vi "MD5 Padding__ogtk.vi"(1 "String":string) -> (0 "MD5 Padded String":string)   [LabVIEW 2015]
panel:
  # "[OpenG VI Tags] ***Do Not Remove***"
  # "MD5 Padding.vi\n\nDerived from the RSA Data Security, Inc. MD5 Message-Digest Algorithm\n\nPlease visit http://www.OpenG.org to learn about the\nOpen Source LabVIEW software movement.\n\nNOTICE -- YOU MUST LEAVE THIS NOTICE IN PLACE.  PER THE TERMS OF THE LICENSE BELOW, YOU MAY SUBLICENSE THIS SOFTWARE \nIN ANY WAY THAT DOES NOT CONFLICT WITH THIS LICENSE.\n\n### BSD License (http://www.opensource.org/licenses/bsd-license.php) Begin ###\n \nCopyright (c) 2004, Enrique Vargas <vargas@visecurity.com>\n\nAll rights reserved.\n\nRedistribution and use in source and binary forms, with or without modification, are permitted provided that the following conditions are met:\n\n    * Redistributions of source code must retain the above copyright notice, this list of conditions and the following disclaimer.\n    * Redistributions in binary form must reproduce the above copyright notice, this list of conditions and the following disclaimer in the \n       documentation and/or other materials provided with the distribution.\n    * Neither the name of SciWare, James Kring, Inc., nor the names of its contributors may be used to endorse or promote products derived \n       from this software without specific prior written permission.\n\nTHIS SOFTWARE IS PROVIDED BY THE COPYRIGHT HOLDERS AND CONTRIBUTORS \"AS IS\" AND ANY EXPRESS OR IMPLIED WARRANTIES, \nINCLUDING, BUT NOT LIMITED TO, THE IMPLIED WARRANTIES OF MERCHANTABILITY AND FITNESS FOR A PARTICULAR PURPOSE ARE \nDISCLAIMED. IN NO EVENT SHALL THE COPYRIGHT OWNER OR CONTRIBUTORS BE LIABLE FOR ANY DIRECT, INDIRECT, INCIDENTAL,\n SPECIAL, EXEMPLARY, OR CONSEQUENTIAL DAMAGES (INCLUDING, BUT NOT LIMITED TO, PROCUREMENT OF SUBSTITUTE GOODS OR \nSERVICES; LOSS OF USE, DATA, OR PROFITS; OR BUSINESS INTERRUPTION) HOWEVER CAUSED AND ON ANY THEORY OF LIABILITY, \nWHETHER IN CONTRACT, STRICT LIABILITY, OR TORT (INCLUDING NEGLIGENCE OR OTHERWISE) ARISING IN ANY WAY OUT OF THE USE \nOF THIS SOFTWARE, EVEN IF ADVISED OF THE POSSIBILITY OF SUCH DAMAGE.\n\n### BSD License End ###"
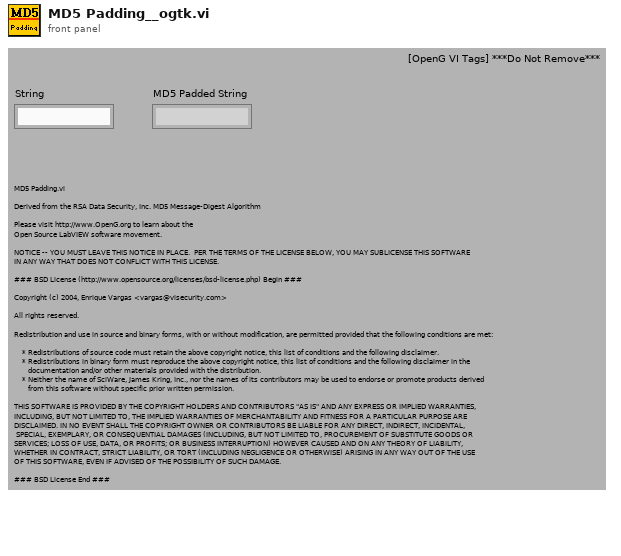
[diagram p1: front panel]
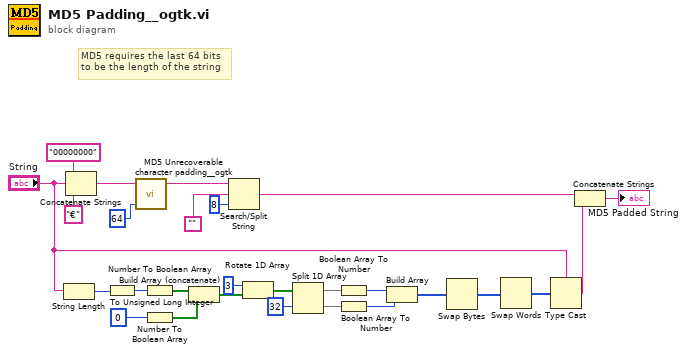
[diagram p0: block diagram]
diagram:
  # "MD5 requires the last 64 bits\nto be the length of the string"
  n1 = String Length(string="String") -> (length=w16:i32)
  n2 = Concatenate Strings("00000000", "String", "€") -> (w25:string)
  n3 = To Unsigned Long Integer(number=w16) -> (unsigned 32bit integer=w13:u32)
  n4 = call "MD5 Unrecoverable character padding__ogtk.vi"("Block Size (16)"=64, "Message"=w25) -> ("Padded message"=w22:string)  [unwired: 3 in]
  n5 = Number To Boolean Array(number=w13) -> (Boolean array=w11:bool[])
  n6 = Number To Boolean Array(number=u32 0 ("length")) -> (Boolean array=w10:bool[])
  n7 = Build Array (concatenate)(w11, w10) -> (w9:bool[])
  n8 = Search/Split String(string=w22, search string/char (-)="", offset (0)=8) -> (match + rest of string=w18:string)  [unwired: 2 out]
  n9 = Rotate 1D Array(1:w9, 2:3 ("n")) -> (0:w7:bool[])
  n10 = Split 1D Array(array=w7, index=32) -> (first subarray=w5:bool[], second subarray=w4:bool[])
  n11 = Boolean Array To Number(Boolean array=w5) -> (number=w3:u32)
  n12 = Boolean Array To Number(Boolean array=w4) -> (number=w2:u32)
  n13 = Build Array(w3, w2) -> (w1:u32[])
  n14 = Swap Bytes(anything=w1) -> (byte swapped=w15:u32[])
  n15 = Swap Words(1:w15) -> (0:w14:u32[])
  n16 = Type Cast(type="String", x=w14) -> (*(type *) &x=w19:string)
  n17 = Concatenate Strings(w18, w19) -> (→"MD5 Padded String":string)
